vi "Create Device Sections.vi"(8 "error in (no error)":errorcluster, 9 "J1939 Monitor Settings":T2 {"Name" format="%.0x"}, 10 "Name":string, 11 "Item Ref in":T1 format="%.0x") -> (0 "error out":errorcluster, 2 "Device Ref out":T1 format="%.0x")   [LabVIEW 2015, in "J1939 Addon Shared.lvlib"]
uses:
  J1939 Addon Shared.lvlib
  Types/Monitor Settings.ctl
  <vilib>/NI Veristand/Custom Device API/Custom Device Item Ref.ctl
  <vilib>/NI Veristand/Custom Device API/Custom Device Channel.ctl
  <vilib>/NI Veristand/Custom Device API/Custom Device Channel Type.ctl
  Constants.vi
  <vilib>/NI VeriStand/Custom Device API/Custom Device API.lvlib
  <vilib>/NI/NI VeriStand Advanced SysDef API/SysDef API/Advanced System Definition.lvlib
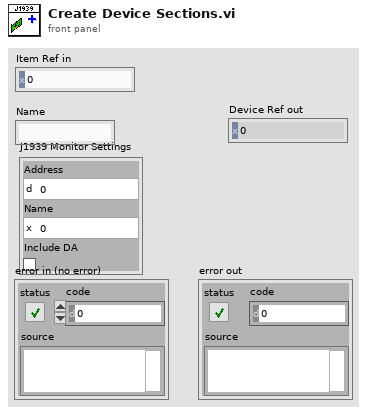
[diagram p1: front panel]
types:
  T1 = typedef "Custom Device API.lvlib/Custom Device Item Ref.ctl" = u64
  T2 = typedef "J1939 Addon Shared.lvlib/Monitor Settings.ctl" = cluster{"Address":u8, "Name":u64, "Include DA":bool}
  T3 = typedef "Custom Device API.lvlib/Custom Device Channel.ctl" = cluster{"Type":T4, "Units":string, "Default Value":dbl, "Faultable":bool, "Scalable":bool}
  T4 = typedef "Custom Device API.lvlib/Custom Device Channel Type.ctl" = enum16{"Input", "Output"}
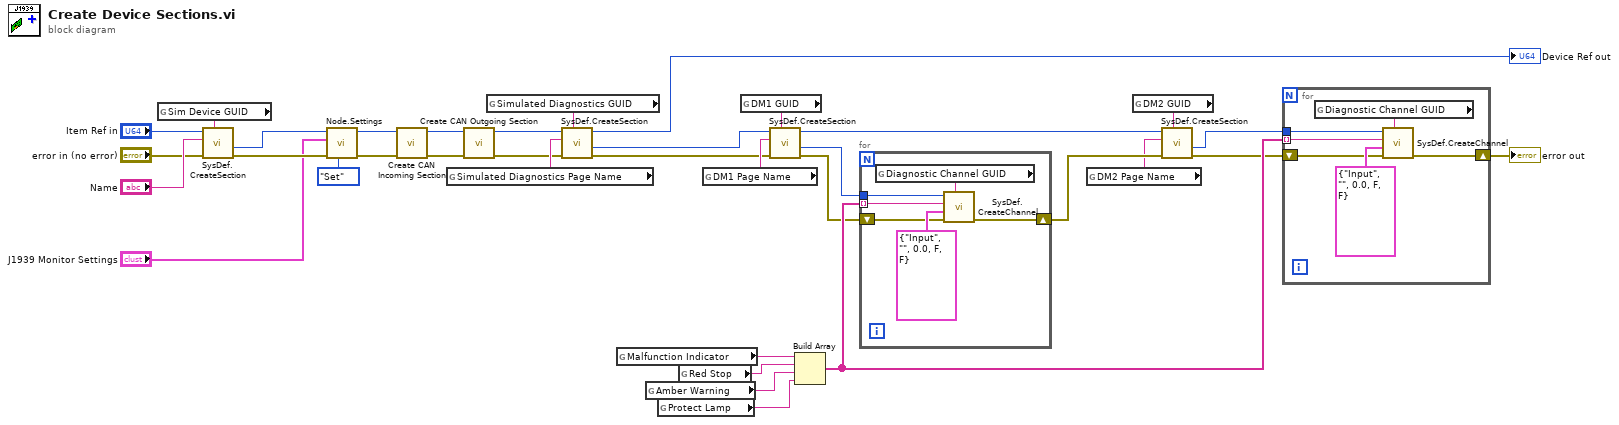
[diagram p0: block diagram]
diagram:
  n1 = global read "Constants.vi" "Sim Device GUID"() -> (w6:string)
  n2 = call <vilib>:"SysDef.CreateSection.vi"("GUID"=w6, "error in (no error)"="error in (no error)", "Name"="Name", "nodeID"="Item Ref in") -> ("error out"=w32:errorcluster, "New NodeID"=w34:u64)  [unwired: 4 in, 2 out]
  n3 = call "Node.Settings.vi"("Action"=enum8{"Get", "Set"}."Set", "error in (no error)"=w32, "Node.Settings"="J1939 Monitor Settings", "Item Ref in"=w34) -> ("error out"=w33:errorcluster, "Item Ref out"=w35:T1)  [unwired: 5 in, 1 out]
  n4 = call "Create CAN Incoming Section.vi"("error in (no error)"=w33, "Device Item Ref in"=w35) -> ("error out"=w4:errorcluster, "Device Item Ref Out"=w5:T1)  [unwired: 8 in]
  n5 = global read "Constants.vi" "Simulated Diagnostics Page Name"() -> (w13:string)
  n6 = call "Create CAN Outgoing Section.vi"("error in (no error)"=w4, "Parent Ref in"=w5) -> ("error out"=w12:errorcluster, "Parent Ref out"=w11:T1)  [unwired: 8 in]
  n7 = global read "Constants.vi" "Simulated Diagnostics GUID"() -> (w10:string)
  n8 = call <vilib>:"SysDef.CreateSection.vi"("GUID"=w10, "error in (no error)"=w12, "Name"=w13, "nodeID"=w11) -> ("error out"=w14:errorcluster, "New NodeID"=w15:u64, "nodeID out"=→"Device Ref out":u64)  [unwired: 4 in, 1 out]
  n9 = global read "Constants.vi" "Malfunction Indicator"() -> (w20:string)
  n10 = global read "Constants.vi" "Amber Warning"() -> (w22:string)
  n11 = global read "Constants.vi" "Protect Lamp"() -> (w23:string)
  n12 = global read "Constants.vi" "Red Stop"() -> (w21:string)
  n13 = global read "Constants.vi" "DM1 Page Name"() -> (w17:string)
  n14 = global read "Constants.vi" "DM1 GUID"() -> (w16:string)
  n15 = call <vilib>:"SysDef.CreateSection.vi"("GUID"=w16, "error in (no error)"=w14, "Name"=w17, "nodeID"=w15) -> ("error out"=w24:errorcluster, "New NodeID"=w26:u64, "nodeID out"=w27:u64)  [unwired: 4 in, 1 out]
  n16 = Build Array(w20, w21, w22, w23) -> (w31:string[])
  n17 = for {
    tunnel: w26 -> [w37]
    shift-right: [w38] -> w25
    shift-left: w24 -> [w39]
    tunnel: w31 -> [w36] mode=indexing
    n18 = global read "Constants.vi" "Diagnostic Channel GUID"() -> (w41:string)
    n19 = call <vilib>:"SysDef.CreateChannel.vi"("GUID"=w41, "error in (no error)"=w39, "Channel"=T3 {"Type"=enum."Input", "Units"="", "Default Value"=0.0, "Faultable"=FALSE, "Scalable"=FALSE}, "Name"=w36, "nodeID"=w37) -> ("error out"=w38:errorcluster)  [unwired: 3 in, 3 out]
  }
  n20 = global read "Constants.vi" "DM2 Page Name"() -> (w18:string)
  n21 = global read "Constants.vi" "DM2 GUID"() -> (w19:string)
  n22 = call <vilib>:"SysDef.CreateSection.vi"("GUID"=w19, "error in (no error)"=w25, "Name"=w18, "nodeID"=w27) -> ("error out"=w29:errorcluster, "New NodeID"=w28:u64)  [unwired: 4 in, 2 out]
  n23 = for {
    tunnel: w28 -> [w43]
    shift-right: [w44] -> w30
    shift-left: w29 -> [w45]
    tunnel: w31 -> [w42] mode=indexing
    n24 = global read "Constants.vi" "Diagnostic Channel GUID"() -> (w47:string)
    n25 = call <vilib>:"SysDef.CreateChannel.vi"("GUID"=w47, "error in (no error)"=w45, "Channel"=T3 {"Type"=enum."Input", "Units"="", "Default Value"=0.0, "Faultable"=FALSE, "Scalable"=FALSE}, "Name"=w42, "nodeID"=w43) -> ("error out"=w44:errorcluster)  [unwired: 3 in, 3 out]
  }
  "error out" <- w30
